vi "Multiply Class Test.vi"() -> ()   [LabVIEW 2021, in "Test Files.lvlib"]
uses:
  Test Files.lvlib
  <vilib>/addons/_JKI Toolkits/Caraya/classes/Test/Test.lvclass
  <vilib>/addons/_JKI Toolkits/Caraya/classes/Assert/Assert.lvclass
  Classes/NumericOperation/NumericOperation.lvclass
  Controls/Test Data Cluster.ctl
  <vilib>/addons/_JKI Toolkits/Caraya/classes/Assert/Assert Equal Value_Variant.vi
panel:
  out "error out":errorcluster
  in  "error in (no error)":errorcluster
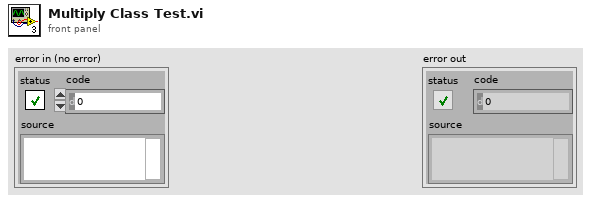
[diagram p1: front panel]
types:
  T1 = typedef "Test Data Cluster.ctl" = cluster{"A":dbl, "B":dbl, "Output":dbl}
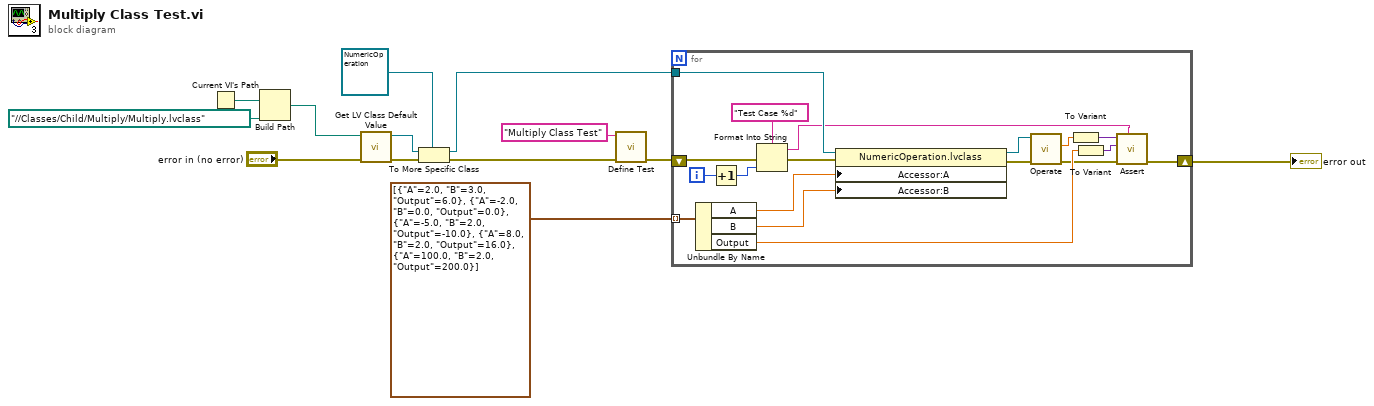
[diagram p0: block diagram]
diagram:
  n1 = Current VI's Path() -> (path=w13:path)
  n2 = Build Path(base path=w13, name or relative path=path "../../Classes/Child/Multiply/Multiply.lvclass") -> (appended path=w11:path)
  n3 = call <vilib>:"Get LV Class Default Value.vi"("error in (no error)"="error in (no error)", "class path"=w11) -> ("error out"=w9:errorcluster, "object"=w4:refnum<class>)  [unwired: 8 in]
  n4 = To More Specific Class(target class=refnum<class "NumericOperation.lvclass"> refnum ("Calculator.lvlib:NumericOperation.lvclass"), reference=w4, error in=w9) -> (specific class reference=w3:refnum<class "NumericOperation.lvclass">, error out=w8:errorcluster)
  n5 = call <vilib>:"Define Test.vi"("error in (no error)"=w8, "Label (VI Title)"="Multiply Class Test") -> ("error out"=w6:errorcluster)  [unwired: 8 in, 1 out]
  n6 = for {
    tunnel: w3 -> [w26]
    tunnel: T1[] [{"A"=2.0, "B"=3.0, "Output"=6.0}, {"A"=-2.0, "B"=0.0, "Output"=0.0}, {"A"=-5.0, "B"=2.0, "Output"=-10.0}, {"A"=8.0, "B"=2.0, "Output"=16.0}, {"A"=100.0, "B"=2.0, "Output"=200.0}] -> [w25] mode=indexing
    shift-right: [w15] -> w1
    shift-left: w6 -> [w31]
    i -> [w30]
    n7 = Unbundle By Name(w25) -> ("A"=w24:dbl, "B"=w23:dbl, "Output"=w17:dbl)
    n8 = Increment(x=w30) -> (x+1=w29:i32)
    n9 = Format Into String(format string="Test Case %d", error in=w31, w29) -> (resulting string=w14:string, error out=w27:errorcluster)  [unwired: 1 in]
    n10 = property class="NumericOperation.lvclass"(reference=w26, error in=w27, "Accessor:A"=w24, "Accessor:B"=w23) -> (reference out=w21:refnum<class "NumericOperation.lvclass">, error out=w22:errorcluster)
    n11 = call-dynamic "Operate.vi"("error in (no error)"=w22, "NumericOperation in"=w21) -> ("error out"=w16:errorcluster, "C"=w20:dbl)  [unwired: 7 in, 1 out]
    n12 = To Variant(anything=w20) -> (Variant=w19:variant)
    n13 = To Variant(anything=w17) -> (Variant=w18:variant)
    n14 = call-poly <vilib>:"Assert.vi"("Label"=w14, "error in (no error)"=w16, "Y"=w18, "X"=w19) -> ("error out"=w15:errorcluster)  [unwired: 6 in, 1 out]
  }
  "error out" <- w1
